vi "firebase.vi"() -> ()   [LabVIEW 2019]
uses:
  <vilib>/httpClient/PUTBuffer.vi
  <vilib>/httpClient/LabVIEWHTTPClient.lvlib
panel:
  in  "stop":bool
  in  "String":string
  in  "mark 2":dbl
  in  "mark 1":dbl
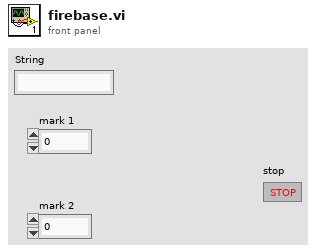
[diagram p1: front panel]
types:
  T1 = typedef "LabVIEWHTTPClient.lvlib/ClientHandle.ctl" = refnum<k1>
  T2 = cluster{"mark 1":dbl, "String":string, "mark 2":dbl}
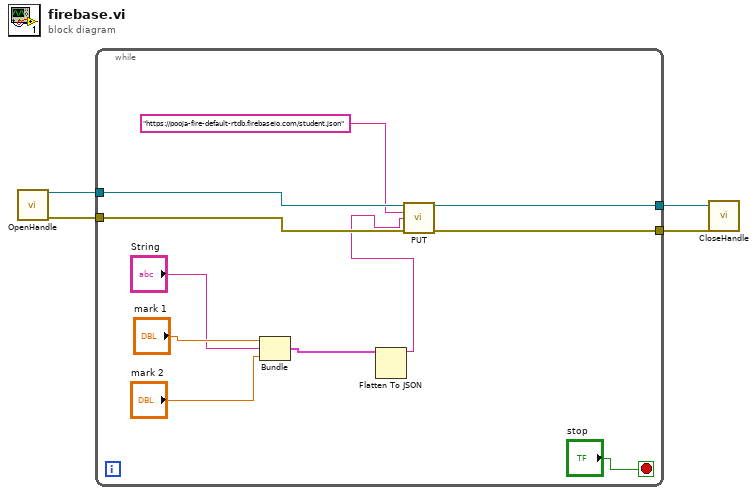
[diagram p0: block diagram]
diagram:
  n1 = call <vilib>:"OpenHandle.vi"() -> ("client handle out"=w4:T1, "error out"=w3:errorcluster)  [unwired: 14 in]
  n2 = while {
    tunnel: w4 -> [w15]
    tunnel: w3 -> [w14]
    tunnel: [w6] -> w2
    tunnel: [w5] -> w1
    stop <- "stop" stop-if-true
    n3 = Bundle("mark 1"="mark 1", "String"="String", "mark 2"="mark 2") -> (w10:T2)  [unwired: 1 in]
    n4 = Flatten To JSON(anything=w10) -> (JSON string=w12:string)  [unwired: 2 in, 1 out]
    n5 = call-poly <vilib>:"PUT.vi"("client handle"=w15, "url"="https://pooja-fire-default-rtdb.firebaseio.com/student.json", "buffer"=w12, "error in (no error)"=w14) -> ("client handle out"=w6:T1, "error out"=w5:errorcluster)  [unwired: 8 in, 2 out]
  }
  n6 = call <vilib>:"CloseHandle.vi"("client handle"=w2, "error in (no error)"=w1) -> ()  [unwired: 13 in, 1 out]
